vi "Sub VI tester.vi"() -> ()   [LabVIEW 2016]
uses:
  type.ctl
panel:
  in  "Datos de entrada":T1={"Current T"=0.0, "Max T"=30.0, "Min T"=10.0, "Warning"="", "Hay peligro?"=FALSE}
  in  "Stop":bool
  out "Warning":string
  out "Hay peligro?":bool
  out "Waveform Chart":dbl(graph)
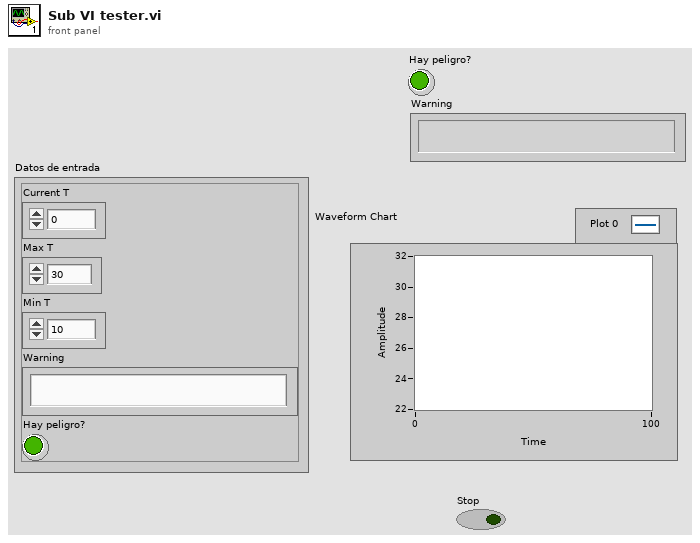
[diagram p1: front panel]
types:
  T1 = typedef "type.ctl" = cluster{"Current T":dbl, "Max T":dbl, "Min T":dbl, "Warning":string, "Hay peligro?":bool}
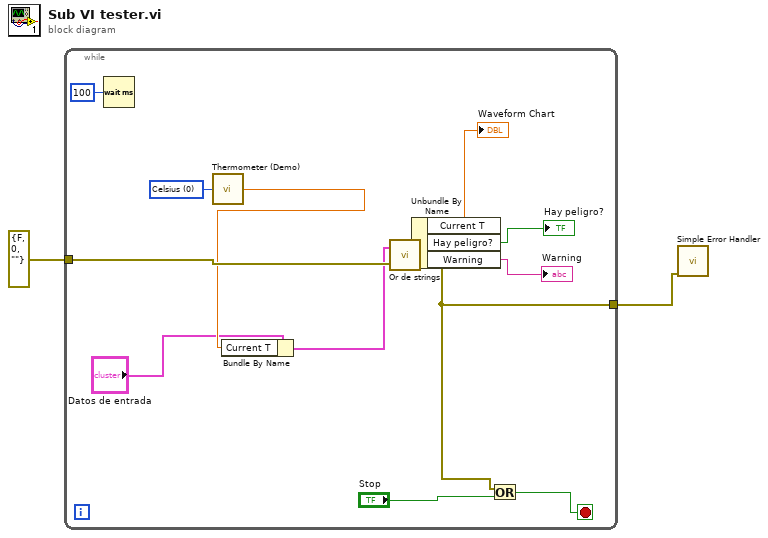
[diagram p0: block diagram]
diagram:
  n1 = while {
    tunnel: errorcluster {"status"=FALSE, "code"=0, "source"=""} ("error constant") -> [w13]
    tunnel: [w10] -> w1
    stop <- w12 stop-if-true
    w15 = u16 0 items=["Celsius", "Fahrenheit"] ("Units (0: Celsius)")
    n2 = Wait (ms)(milliseconds to wait=u32 100) -> ()  [unwired: 1 out]
    n3 = call "Thermometer (Demo).vi"("Units (0: Celsius)"=w15) -> ("Temperature Value"=w9:dbl)
    n4 = Bundle By Name(cluster="Datos de entrada", "Current T"=w9) -> (w8:T1)
    n5 = call "Or de strings.vi"("Error In"=w13, "Datos de entrada"=w8) -> ("Error Out"=w10:errorcluster, "Datos de salida"=w6:T1)
    n6 = Unbundle By Name(w6) -> ("Current T"=→"Waveform Chart":dbl, "Hay peligro?"=→"Hay peligro?":bool, "Warning"=→"Warning":string)
    n7 = Or(x=w10, y="Stop") -> (x .or. y?=w12:bool)
  }
  n8 = call <vilib>:"Simple Error Handler.vi"("error in (no error)"=w1) -> ()  [unwired: 4 in, 5 out]
